vi "kD2A FPGA.vi"(6 "Timeout":i32=40000000, 9 "DIO Port Selection":T1={"Controller Port CLK"="Connector0/DIO1", "Controller Port SIG"="Connector0/DIO1", "DA Port CLK"="Connector0/DIO1", "DA Port SIG"="Connector0/DIO1"}, 11 "FIFO Out":refnum<k21>="kD2A Board Fifo") -> ()   [LabVIEW 2011, in "kevLib2011.lvlib"]
uses:
  kevLib2011.lvlib
  KD2A Port Sel.ctl
  <vilib>/rvi/DataTransferAndStorage/Container/Common/niFpgaContainerExecOnDevCompGetState.vi
  <vilib>/rvi/FIFO/Fifo_Resource/nirvififoEmulationSetSize.vi
  <vilib>/rvi/DataTransferAndStorage/Container/Common/niFpgaContainerGetUniqueNameForEmu.vi
  <vilib>/rvi/interface/RandomDataEmulation/nirviRandomDataFPGAFIFO.vi
  <vilib>/rvi/interface/RandomDataEmulation/niFpgaRandomDataHandleErrors.vi
  <vilib>/rvi/eio/common/nirviEmuReportErrorAndStop.vi
  <vilib>/rvi/DataTransferAndStorage/Container/XNode/niFpgaContainer.xnode
  <vilib>/rvi/FIFO/Fifo_Resource/niFpgaFifoEmulationRefIn.vi
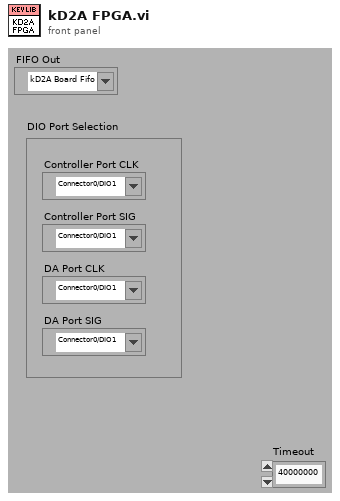
[diagram p1: front panel]
types:
  T1 = typedef "kevLib2011.lvlib/KD2A Port Sel.ctl" = cluster{"Controller Port CLK":refnum<k21>, "Controller Port SIG":refnum<k21>, "DA Port CLK":refnum<k21>, "DA Port SIG":refnum<k21>}
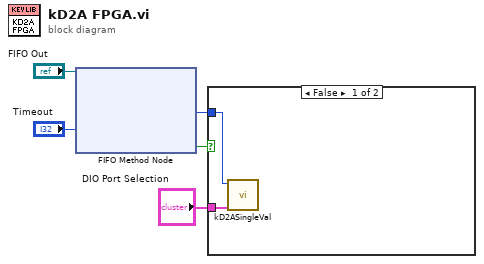
[diagram p0: block diagram]
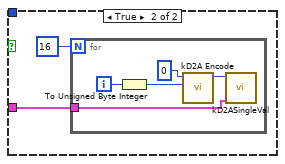
[diagram p2: hidden frame]
diagram:
  n1 = xnode ("FIFO Method Node")("Timeout"="Timeout", "FIFO In"="FIFO Out") -> ("Element"=w2:u16, "Timed Out?"=w3:bool)  [unwired: 1 out]
  n2 = case shown="False" w3 {
    tunnel: w2 -> [w7 _]
    tunnel: "DIO Port Selection" -> [w6 w8]
    frame False {
      n3 = call "kD2ASingleVal.vi"("DIO Port Selection"=w6, "Single Input Element"=w7) -> ()  [unwired: 10 in]
    }
    frame True {
      n4 = for {
        N: 16 -> [_]
        tunnel: w8 -> [w10]
        i -> [w14]
        n5 = To Unsigned Byte Integer(number=w14) -> (unsigned 8bit integer=w13:u8)
        n6 = call "kD2A Encode.vi"("Position"=w13, "Value"=i16 0) -> ("Coded Output"=w11:u16)  [unwired: 9 in]
        n7 = call "kD2ASingleVal.vi"("DIO Port Selection"=w10, "Single Input Element"=w11) -> ()  [unwired: 10 in]
      }
    }
  }
